vi "Remove Subtree Meta.vi"(8 "error in (no error)":errorcluster, 10 "Config":refnum<class "Config Manager.lvclass">, 11 "Config Storage in":refnum<class "Config Storage.lvclass">) -> (0 "error out":errorcluster, 3 "Config Storage out":refnum<class "Config Storage.lvclass">)   [LabVIEW 2020, in "CDM-Config.lvlib" / "Config Storage.lvclass"]
uses:
  Config Storage.lvclass
  Config Manager/Config Manager.lvclass
  Config Storage.lvclass/Config Storage.ctl
  Config Element/Config Element.lvclass
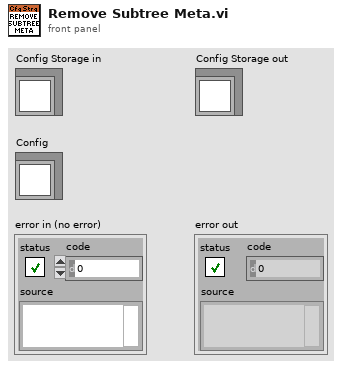
[diagram p1: front panel]
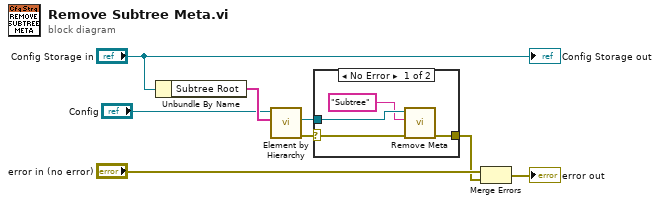
[diagram p0: block diagram]
diagram:
  n1 = Unbundle By Name("Config Storage in") -> ("Subtree Root"=w6:string[])
  n2 = call "Element by Hierarchy.vi"("Hierarchy"=w6, "Config Manager in"="Config") -> ("error out"=w4:errorcluster, "Config Element"=w3:refnum<class "Config Element.lvclass">)  [unwired: 7 in, 1 out]
  n3 = case shown="No Error" w4 {
    selector: w4 -> [w11 w13]
    tunnel: w3 -> [w12 _]
    tunnel: [w9 w13] -> w1
    frame No Error {
      n4 = call "Remove Meta.vi"("error in (no error)"=w11, "Meta Name"="Subtree", "Config Element in"=w12) -> ("error out"=w9:errorcluster)  [unwired: 6 in, 2 out]
    }
    frame Error {
    }
  }
  n5 = Merge Errors("error in (no error)", w1) -> (→"error out":errorcluster)
  "Config Storage out" <- "Config Storage in"
